vi "movement_control_panel.vi"() -> ()   [LabVIEW 2014]
uses:
  <vilib>/Motion/Express/_s/nimc.ex.read.readExecutionData.axis.vi
  <vilib>/Motion/BlockNode/FB.NIMotion.xnode
panel:
  out "Delay Over?":bool
  in  "Position data":path
  in  "Return to position":bool
  in  "Save position":bool
  out "Single Plot (Array of X,Y Pairs)":cluster{u32[], dbl[]}(graph)
  in  "Injury Duration (ms)":dbl=30.0
  in  "Injury (mm)":dbl=2.0
  in  "Near Bottom":bool
  in  "Top (disconnect)":bool
  in  "+1 mm":bool
  in  "+1/10 mm":bool
  in  "-1 mm":bool
  in  "-1/10 mm":bool
  in  "INJURE":bool
  out "Current Position (dum)":dbl
  in  "stop":bool
  # "Raise the platform\n(Negative displacement)"
  # "Lower the platform\n(Positive displacement)"
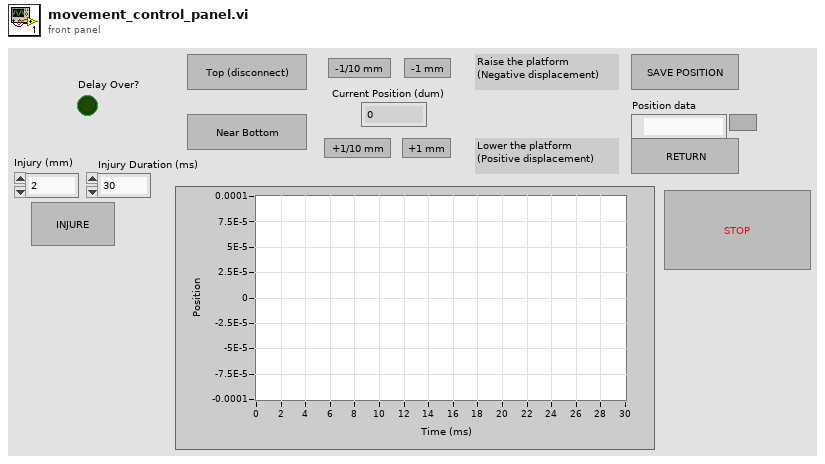
[diagram p1: front panel]
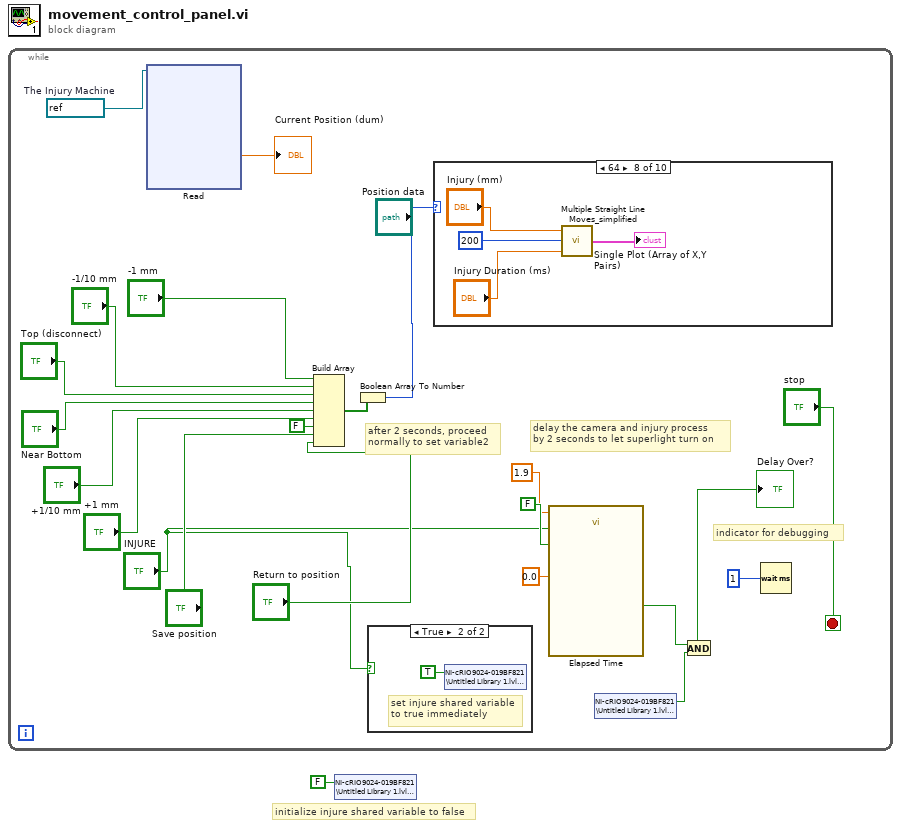
[diagram p0: block diagram]
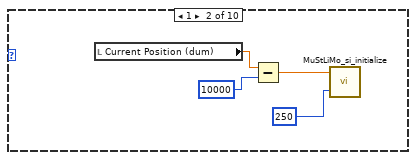
[diagram p4: hidden frame]
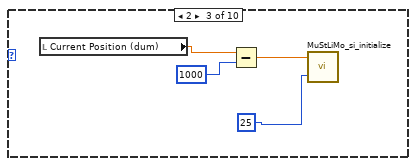
[diagram p5: hidden frame]
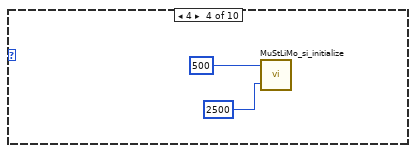
[diagram p6: hidden frame]
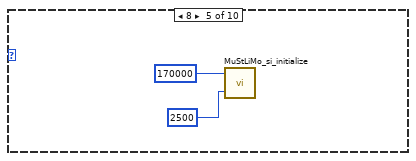
[diagram p7: hidden frame]
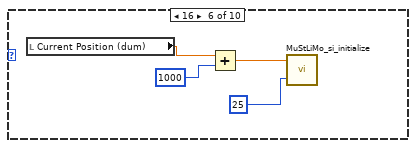
[diagram p8: hidden frame]
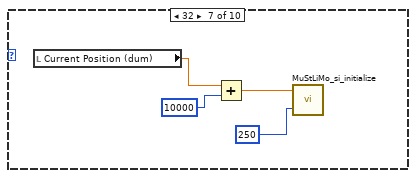
[diagram p9: hidden frame]
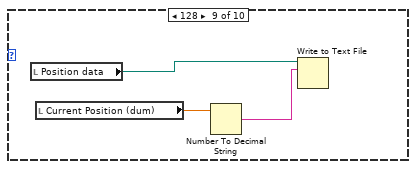
[diagram p10: hidden frame]
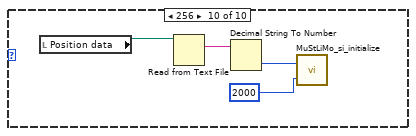
[diagram p11: hidden frame]
diagram:
  # "initialize injure shared variable to false"
  n1 = while {
    stop <- "stop" stop-if-true
    w22 = refnum<k21> "Axis 1"  # The Injury Machine
    # "indicator for debugging"
    # "after 2 seconds, proceed \nnormally to set variable2"
    # "delay the camera and injury process \nby 2 seconds to let superlight turn on"
    n2 = xnode ("Read")("resource"=w22) -> ("position"=→"Current Position (dum)":dbl)  [unwired: 1 in, 6 out]
    n3 = Build Array("-1 mm", "-1/10 mm", "Top (disconnect)", "Near Bottom", "+1/10 mm", "+1 mm", FALSE ("element"), "Save position", "Return to position") -> (w14:bool[])
    n4 = Boolean Array To Number(Boolean array=w14) -> (number=w13:u32)
    n5 = case shown="True" "INJURE" {
      frame False {
      }
      frame True {
        # "set injure shared variable\nto true immediately"
        n6 = shared-variable "NI-cRIO9024-019BF821\\Untitled Library 1.lvlib\\INJURE"(TRUE ("INJURE")) -> ()  [unwired: 1 in, 1 out]
      }
    }
    n7 = case shown="64" w13 {
      frame 0, Default {
      }
      frame 1 {
        n8 = local read "Current Position (dum)"() -> (w28:dbl)
        n9 = Subtract(x=w28, y=10000) -> (x-y=w26:dbl)
        n10 = call "MuStLiMo_si_initialize.vi"("Target Pulse Duration (ms)"=250, "Target Position (decimicrons)"=w26) -> ()  [unwired: 1 in]
      }
      frame 2 {
        n11 = local read "Current Position (dum)"() -> (w29:dbl)
        n12 = Subtract(x=w29, y=1000) -> (x-y=w32:dbl)
        n13 = call "MuStLiMo_si_initialize.vi"("Target Pulse Duration (ms)"=25, "Target Position (decimicrons)"=w32) -> ()  [unwired: 1 in]
      }
      frame 4 {
        n14 = call "MuStLiMo_si_initialize.vi"("Target Pulse Duration (ms)"=2500, "Target Position (decimicrons)"=500) -> ()  [unwired: 1 in]
      }
      frame 8 {
        n15 = call "MuStLiMo_si_initialize.vi"("Target Pulse Duration (ms)"=2500, "Target Position (decimicrons)"=170000) -> ()  [unwired: 1 in]
      }
      frame 16 {
        n16 = local read "Current Position (dum)"() -> (w37:dbl)
        n17 = Add(x=w37, y=1000) -> (x+y=w39:dbl)
        n18 = call "MuStLiMo_si_initialize.vi"("Target Pulse Duration (ms)"=25, "Target Position (decimicrons)"=w39) -> ()  [unwired: 1 in]
      }
      frame 32 {
        n19 = local read "Current Position (dum)"() -> (w41:dbl)
        n20 = Add(x=w41, y=10000) -> (x+y=w43:dbl)
        n21 = call "MuStLiMo_si_initialize.vi"("Target Pulse Duration (ms)"=250, "Target Position (decimicrons)"=w43) -> ()  [unwired: 1 in]
      }
      frame 64 {
        n22 = call "Multiple Straight Line Moves_simplified.vi"("Target Pulse Duration (ms)"="Injury Duration (ms)", "Sync lag"=200, "Target Peak Displacement (mm)"="Injury (mm)") -> ("Single Plot (Array of X,Y Pairs)"=→"Single Plot (Array of X,Y Pairs)":cluster{u32[], dbl[]})
      }
      frame 128 {
        n23 = local read "Position data"() -> (w49:path)
        n24 = local read "Current Position (dum)"() -> (w51:dbl)
        n25 = Number To Decimal String(number=w51) -> (decimal integer string=w50:string)  [unwired: 1 in]
        n26 = Write to Text File(file (use dialog)=w49, text=w50) -> ()  [unwired: 2 in, 3 out]
      }
      frame 256 {
        n27 = local read "Position data"() -> (w55:path)
        n28 = Read from Text File(file (use dialog)=w55) -> (text=w54:string)  [unwired: 3 in, 3 out]
        n29 = Decimal String To Number(string=w54) -> (number=w53:i32)  [unwired: 2 in, 1 out]
        n30 = call "MuStLiMo_si_initialize.vi"("Target Pulse Duration (ms)"=2000, "Target Position (decimicrons)"=w53) -> ()  [unwired: 1 in]
      }
    }
    n31 = call "Elapsed Time"("Time Target (s)"=1.9, "Reset"="INJURE", "Auto Reset"=FALSE, "Set Start Time (s)"=0.0) -> ("Time has Elapsed"=w6:bool)  [unwired: 8 in, 7 out]
    n32 = shared-variable "NI-cRIO9024-019BF821\\Untitled Library 1.lvlib\\INJURE"() -> (w5:bool)  [unwired: 1 in, 1 out]
    n33 = And(x=w6, y=w5) -> (x .and. y?=→"Delay Over?":bool)
    n34 = Wait (ms)(milliseconds to wait=1) -> ()  [unwired: 1 out]
  }
  n35 = shared-variable "NI-cRIO9024-019BF821\\Untitled Library 1.lvlib\\INJURE"(FALSE ("INJURE")) -> ()  [unwired: 1 in, 1 out]
